vi "sio DTR.vi"(8 "mode":i32, 11 "port":i32) -> (3 "port":i32)   [LabVIEW 2015, in "PCOMM.lvlib"]
doc: "int WINAPI sio_DTR(int port, int mode);\nmode=1:DTR ON\nmode=0:DTR OFF"
uses:
  PCOMM.lvlib
  PCOMM.DLL
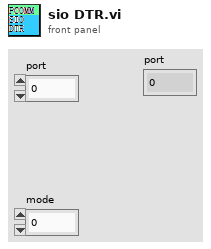
[diagram p1: front panel]
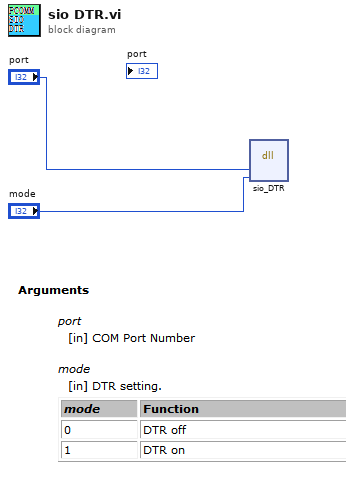
[diagram p0: block diagram]
diagram:
  n1 = dll-call lib="PTH2^abs EDesktopLabview串口助手串口助手2.0Ing10_v3.2.0SubVIpcomm库PCOMM.*" fn="sio_DTR"("port"="port", "mode"="mode") -> ()  [unwired: 6 in, 2 out]
